vi "Enter Return Data.vi"(8 "error in (no error)":errorcluster, 10 "Return Data":string, 11 "DataGrid in":refnum<class "DataGrid.lvclass">) -> (0 "error out":errorcluster, 3 "DataGrid out":refnum<class "DataGrid.lvclass">)   [LabVIEW 2017, in "DataGrid.lvclass"]
uses:
  DataGrid.lvclass
  C:/Program Files (x86)/National Instruments/LabVIEW 2017/vi.lib/QSI/QControls/QControl Classes/MulticolumnListbox/MulticolumnListbox.lvclass
  Read Current Edit Position.vi
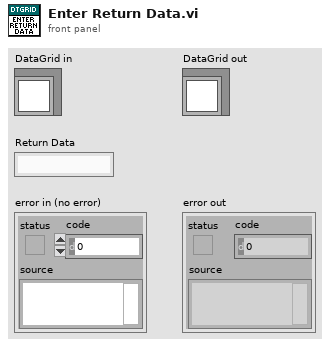
[diagram p1: front panel]
types:
  T1 = typedef "LVRowAndColumnTypeDef.ctl" = cluster{"Row":i32, "Column":i32}
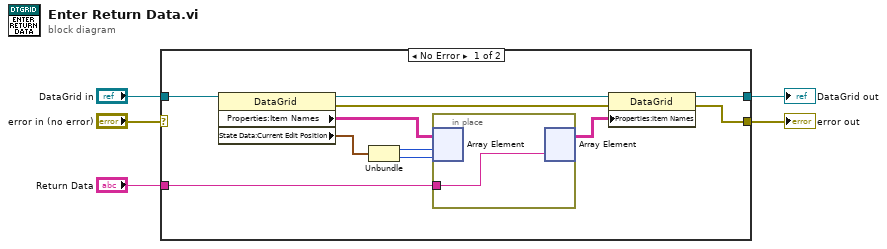
[diagram p0: block diagram]
diagram:
  n1 = case shown="No Error" "error in (no error)" {
    selector: "error in (no error)" -> [_ w19]
    tunnel: [w6 w19] -> w4
    tunnel: [w9 w18] -> w2
    tunnel: "DataGrid in" -> [w16 w18]
    tunnel: "Return Data" -> [w10 _]
    frame No Error {
      n2 = property class="DataGrid"(reference=w16) -> (reference out=w15:refnum<class "DataGrid.lvclass">, error out=w7:errorcluster, "Properties:Item Names"=w14:string[][], "State Data:Current Edit Position"=w13:T1)  [unwired: 1 in]
      n3 = Unbundle(w13) -> ("Row"=w12:i32, "Column"=w11:i32)
      n4 = in-place {
        in-place-border: w10 -> [w17]
        n5 = in-place-array #1(w14, w12, w11) -> ()  [unwired: 1 out]
        n6 = in-place-array #1(w17) -> (w8:string[][])  [unwired: 2 out]
      }
      n7 = property class="DataGrid"(reference=w15, error in=w7, "Properties:Item Names"=w8) -> (reference out=w9:refnum<class "DataGrid.lvclass">, error out=w6:errorcluster)
    }
    frame Error {
    }
  }
  "error out" <- w4
  "DataGrid out" <- w2
